vi "Reset Mutation History.vi"(11 "LabVIEW Object":refnum<class>) -> (3 "size(s)":i32)   [LabVIEW 2015, in "Utility.lvlib"]
uses:
  Utility.lvlib
  <vilib>/Utility/EditLVLibs/LVClass/Mutation History.ctl
  <vilib>/Utility/EditLVLibs/LVClass/Mutation Record.ctl
  <vilib>/Utility/EditLVLibs/LibVersion.ctl
  <vilib>/Utility/EditLVLibs/Edit LVLibs.lvlib
panel:
  out "Mutation History Before":T1 {"LabVIEW Version" format="%.0x"}
  out "Mutation History After":T1 {"LabVIEW Version" format="%.0x"}
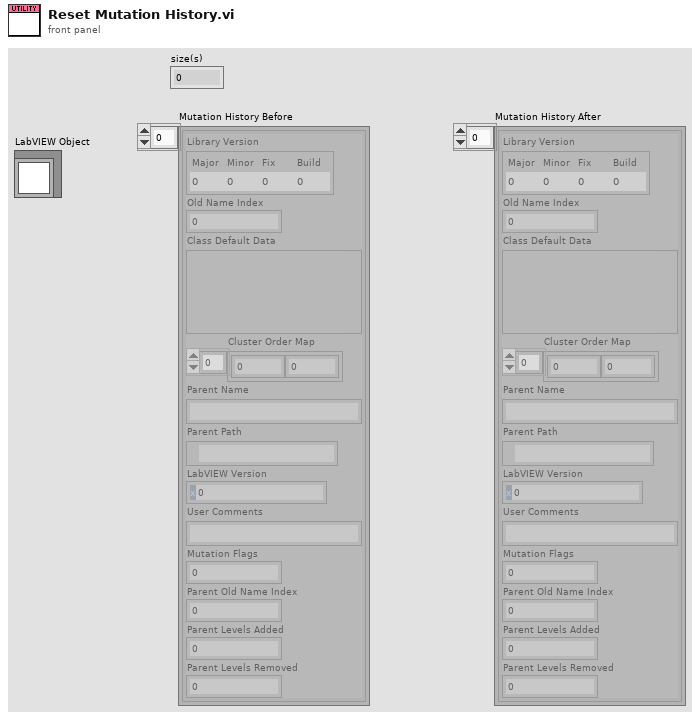
[diagram p1: front panel]
types:
  T1 = typedef "Edit LVLibs.lvlib/Mutation History.ctl" = T2[]
  T2 = typedef "Edit LVLibs.lvlib/Mutation Record.ctl" = cluster{"Library Version":T3, "Old Name Index":u8, "Class Default Data":variant, "Cluster Order Map":u32[], "Parent Name":string, "Parent Path":path, "LabVIEW Version":u32, "User Comments":string, "Mutation Flags":u8, "Parent Old Name Index":u8, "Parent Levels Added":u16, "Parent Levels Removed":u16}
  T3 = typedef "Edit LVLibs.lvlib/LibVersion.ctl" = cluster{"Major":u16, "Minor":u16, "Fix":u16, "Build":u16}
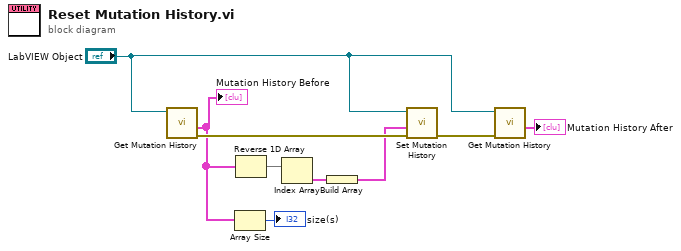
[diagram p0: block diagram]
diagram:
  n1 = call <vilib>:"Get Mutation History.vi"("Input object"="LabVIEW Object") -> ("error out"=w9:errorcluster, "Mutation History"=w2:T1)  [unwired: 7 in]
  "Mutation History Before" <- w2
  n2 = Array Size(array=w2) -> (size(s)=→"size(s)":i32)
  n3 = Reverse 1D Array(array=w2) -> (reversed array=w6:T1)
  n4 = Index Array(array=w6) -> (element=w5:T2)  [unwired: 1 in]
  n5 = Build Array(w5) -> (w4:T2[])
  n6 = call <vilib>:"Set Mutation History.vi"("error in"=w9, "Mutation History"=w4, "Input object"="LabVIEW Object") -> ("error out"=w8:errorcluster)  [unwired: 8 in]
  n7 = call <vilib>:"Get Mutation History.vi"("error in"=w8, "Input object"="LabVIEW Object") -> ("Mutation History"=→"Mutation History After":T1)  [unwired: 6 in, 1 out]
